vi "REF_LEV.vi"(0 "Session In":refnum<visa-resource-name>="GPIB0::16::INSTR", 5 "RefLvl":dbl format="%#_13g", 7 "RefLvl":string, 11 "error in":errorcluster {"code" format="%.0x"}, 12 "RO (T)":bool) -> (4 "Session Out":refnum<visa-resource-name>, 8 "Read":dbl, 14 "Ref LVL coerced (T)":bool, 15 "error out":errorcluster {"code" format="%.0x"})   [LabVIEW 2018]
doc: "Launches the Instrument I/O Assistant, which you can use to communicate with message-based instruments and graphically parse the response. For example you can communicate with an instrument that uses a serial, Ethernet, or GPIB interface."
panel:
  in  "Timeout":u32=3000
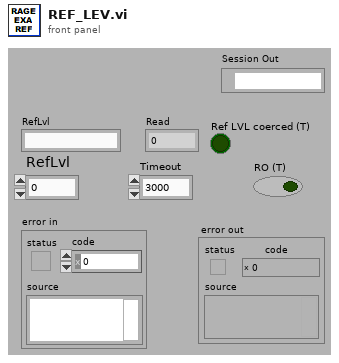
[diagram p1: front panel]
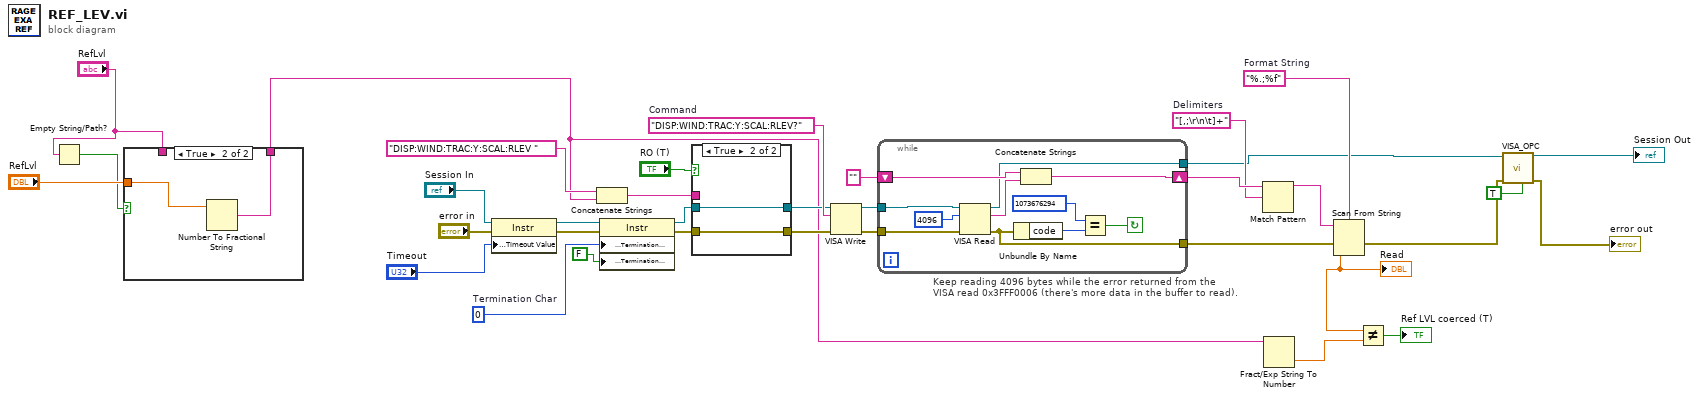
[diagram p0: block diagram]
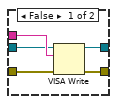
[diagram p3: hidden frame]
diagram:
  w16 = "[,;\r\n\t]+"  # Delimiters
  w17 = "%.;%f"  # Format String
  w20 = "DISP:WIND:TRAC:Y:SCAL:RLEV?"  # Command
  w30 = u8 0  # Termination Char
  # "Keep reading 4096 bytes while the error returned from the\nVISA read 0x3FFF0006 (there's more data in the buffer to read)."
  n1 = Empty String/Path?(string/path="RefLvl") -> (empty?=w8:bool)
  n2 = case shown="True" w8 {
    tunnel: "RefLvl" -> [_ w38]
    tunnel: [w36 w37] -> w7
    tunnel: "RefLvl" -> [w36 _]
    frame False {
    }
    frame True {
      n3 = Number To Fractional String(number=w38) -> (F-format string=w37:string)  [unwired: 3 in]
    }
  }
  n4 = property class="Instr"(reference="Session In", error in="error in", "General Settings:Timeout Value"="Timeout") -> (reference out=w29:refnum<visa-resource-name>, error out=w32:errorcluster)
  n5 = Concatenate Strings("DISP:WIND:TRAC:Y:SCAL:RLEV " ("staticText"), w7) -> (w25:string)
  n6 = property class="Instr"(reference=w29, error in=w32, "Message Based Settings:Termination Character"=w30, "Message Based Settings:Termination Character Enable"=FALSE ("enable")) -> (reference out=w15:refnum<visa-resource-name>, error out=w31:errorcluster)
  n7 = case shown="True" "RO (T)" {
    tunnel: w31 -> [w43 w44]
    tunnel: [w42 w44] -> w26
    tunnel: w25 -> [w41 _]
    tunnel: w15 -> [w40 w45]
    tunnel: [w39 w45] -> w14
    frame False {
      n8 = VISA Write(VISA resource name=w40, write buffer=w41, error in (no error)=w43) -> (VISA resource name out=w39:refnum<visa-resource-name>, error out=w42:errorcluster)  [unwired: 1 out]
    }
    frame True {
    }
  }
  n9 = VISA Write(VISA resource name=w14, write buffer=w20, error in (no error)=w26) -> (VISA resource name out=w24:refnum<visa-resource-name>, error out=w23:errorcluster)  [unwired: 1 out]
  n10 = while {
    tunnel: w24 -> [w53]
    shift-right: [w47] -> w19
    shift-left: "" -> [w52]
    tunnel: w23 -> [w50]
    tunnel: [w49] -> w22
    tunnel: [w46] -> w2
    stop <- w48 continue-if-true
    n11 = VISA Read(VISA resource name=w53, byte count=u32 4096 ("byte count (0)"), error in (no error)=w50) -> (VISA resource name out=w46:refnum<visa-resource-name>, read buffer=w51:string, error out=w49:errorcluster)  [unwired: 1 out]
    n12 = Unbundle By Name(w49) -> ("code"=w55:i32)
    n13 = Concatenate Strings(w52, w51) -> (w47:string)
    n14 = Equal?(x=1073676294, y=w55) -> (x = y?=w48:bool)
  }
  n15 = Match Pattern(string=w19, regular expression=w16) -> (before substring=w18:string)  [unwired: 1 in, 3 out]
  n16 = Fract/Exp String To Number(string=w7) -> (number=w11:dbl)  [unwired: 3 in, 1 out]
  n17 = Scan From String(format string=w17, input string=w18, error in=w22) -> (error out=w5:errorcluster, output 1=w12:dbl)  [unwired: 2 in, 2 out]
  "Read" <- w12
  n18 = Not Equal?(x=w12, y=w11) -> (x != y?=→"Ref LVL coerced (T)":bool)
  n19 = call "VISA_OPC.vi"("OPC(T)"=TRUE ("OPC?(T)"), "error in"=w5, "Session In"=w2) -> ("error out"=→"error out":errorcluster, "Session Out"=→"Session Out":refnum<visa-resource-name>)  [unwired: 6 in, 1 out]
